vi "update_xy_graph.vi"(8 "error in (no error)":errorcluster, 10 "xy_data":cluster{dbl[], dbl[]}[](array[cluster]), 11 "events":T1) -> (0 "error out":errorcluster, 3 "events_out":T1)   [LabVIEW 2015]
uses:
  swabian_events_tdef.ctl
  update_chart_tdef.ctl
  channel_data_tdef.ctl
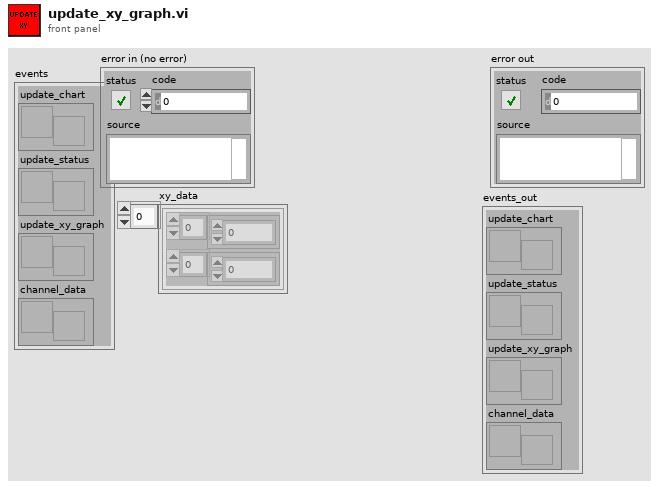
[diagram p1: front panel]
types:
  T1 = typedef "swabian_events_tdef.ctl" = cluster{"update_chart":refnum<user-event>, "update_status":refnum<user-event>, "update_xy_graph":refnum<user-event>, "channel_data":refnum<user-event>}
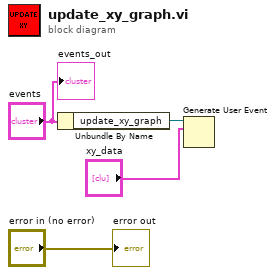
[diagram p0: block diagram]
diagram:
  n1 = Unbundle By Name("events") -> ("update_xy_graph"=w3:refnum<user-event>)
  n2 = Generate User Event(user event=w3, event data cluster="xy_data") -> ()  [unwired: 2 in, 2 out]
  "error out" <- "error in (no error)"
  "events_out" <- "events"
